vi "Mapping Data Plot.vi"() -> ()   [LabVIEW 2012]
uses:
  <vilib>/Utility/miscctls.llb/LVPointDoubleTypeDef.ctl
  <vilib>/Utility/file.llb/Write To Spreadsheet File (DBL).vi
panel:
  in  "Write to file":bool
  out "Counts under curve":dbl[][](array[numeric])=[[0.0, 105.0, 108.0, 96.0, 96.0, 91.0, 85.0], [0.0, 133.0, 105.0, 97.0, 115.0, 96.0, 86.0], [0.0, 257.0, 244.0, 227.0, 195.0, 194.0, 94.0], [0.0, 255.0, 253.0, 258.0, 293.0, 296.0, 96.0], [0.0, 125.0, 160.0, 164.0, 196.0, 206.0, 83.0], [0.0, 107.0, 106.0, 102.0, 94.0, 103.0, 99.0]]
  in  "Cursor.Cursor Position 2":T1
  in  "peak centerRcm-1":dbl=519.0
  in  "peak widthRcm-1":dbl=8.0
  out "error out":errorcluster
  out "Raman Map":dbl[][](graph)
  in  "stop":bool
  out "plot graph":cluster{"Y":dbl[], "Y":dbl[]}[](graph)
  in  "Path":path=path "E:/Documents/lab/Maps"
  in  "2 Letter File Name":string="QS"
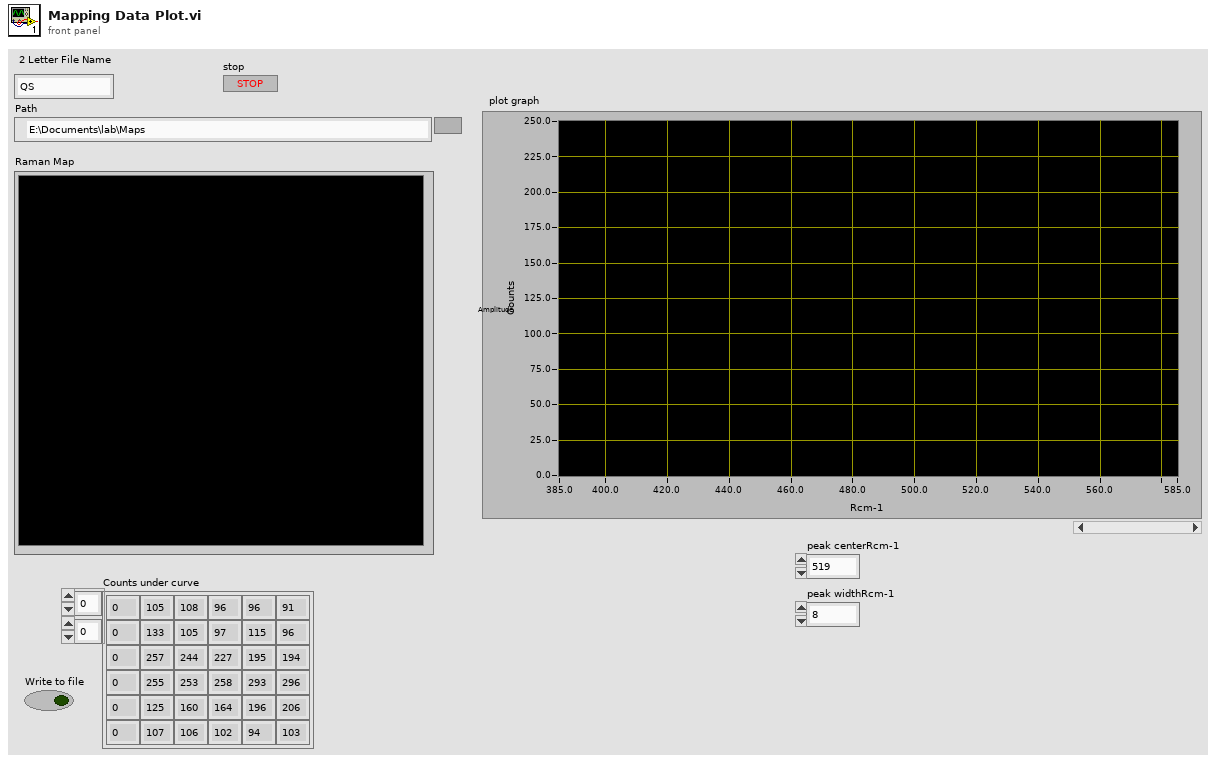
[diagram p1: front panel]
types:
  T1 = typedef "LVPointDoubleTypeDef.ctl" = cluster{"X":dbl, "Y":dbl}
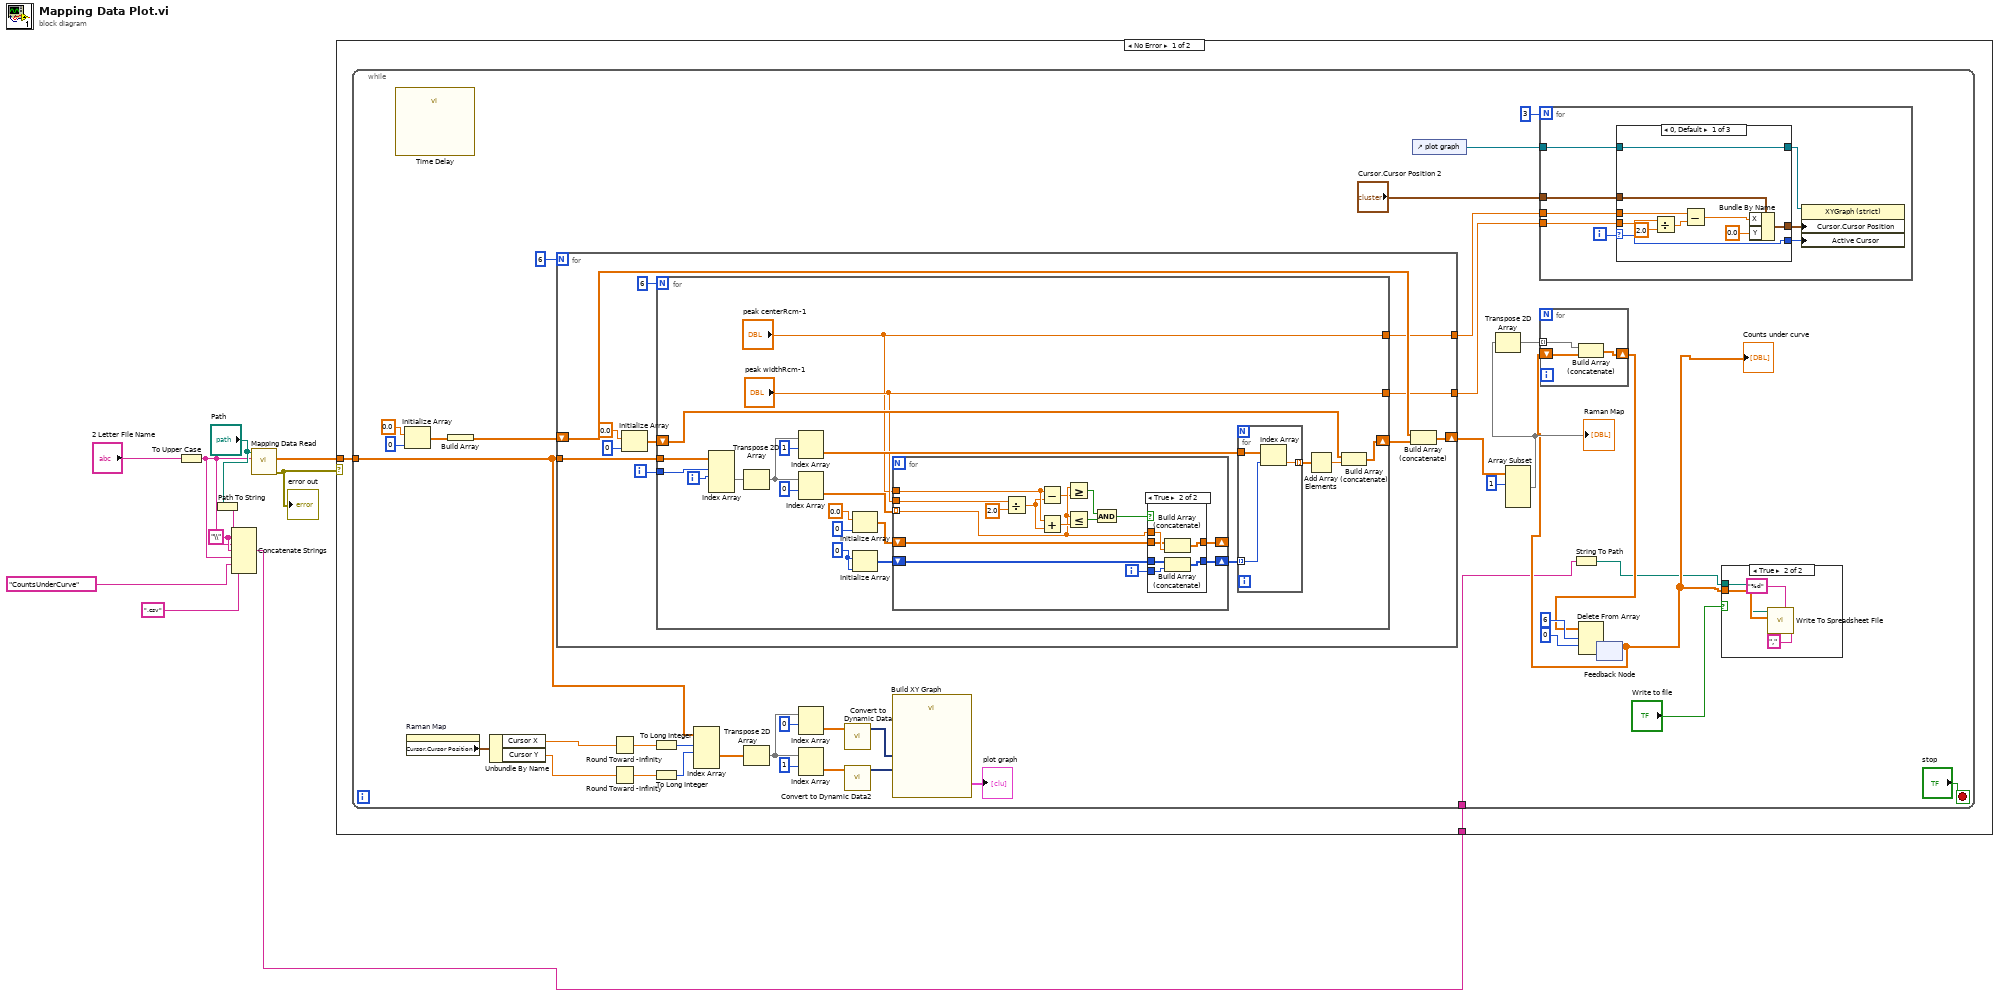
[diagram p0: block diagram]
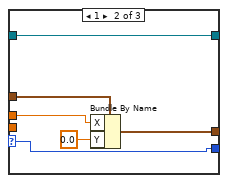
[diagram p3: hidden frame]
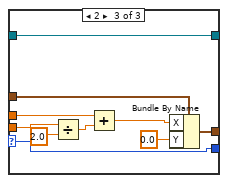
[diagram p4: hidden frame]
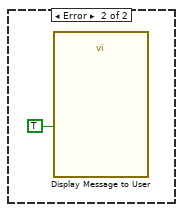
[diagram p6: hidden frame]
diagram:
  w5 = "\\" ("string")
  n1 = To Upper Case(1:"2 Letter File Name") -> (0:w3:string)
  n2 = Path To String(path="Path") -> (string=w6:string)
  n3 = Concatenate Strings(w6, w5, w3, w5, w3, "CountsUnderCurve" ("string"), ".csv") -> (w4:string)
  n4 = call "Mapping Data Read.vi"("Small File name"=w3, "Path"="Path") -> ("error out"=w9:errorcluster, "all rows"=w10:dbl[][][][])  [unwired: 8 in]
  "error out" <- w9
  n5 = case shown="No Error" w9 {
    tunnel: w10 -> [w12 _]
    tunnel: w4 -> [w11 _]
    frame No Error {
      n6 = while {
        tunnel: w12 -> [w43]
        tunnel: w11 -> [w15]
        stop <- "stop" stop-if-true
        n7 = call "Time Delay"() -> ()  [unwired: 11 in, 1 out]
        n8 = Initialize Array(0.0 ("element"), 0 ("dimension size")) -> (w39:dbl[])
        n9 = property on="Raman Map" class="IntGraph (strict)"() -> ("Cursor.Cursor Position"=w30:T1)  [unwired: 2 in, 2 out]
        n10 = Build Array(w39) -> (w38:dbl[][])
        n11 = Unbundle By Name(w30) -> ("Cursor X"=w22:dbl, "Cursor Y"=w29:dbl)
        n12 = for {
          N: 6 -> [_]
          tunnel: w43 -> [w104]
          shift-right: [w96] -> w24
          shift-left: w38 -> [w97]
          tunnel: [w95] -> w36
          tunnel: [w94] -> w32
          i -> [w103]
          n13 = Initialize Array(0.0 ("element"), 0 ("dimension size")) -> (w99:dbl[])
          n14 = for {
            N: 6 -> [_]
            tunnel: w104 -> [w116]
            tunnel: w103 -> [w115]
            shift-right: [w108] -> w98
            shift-left: w99 -> [w107]
            tunnel: ["peak centerRcm-1"] -> w95
            tunnel: ["peak widthRcm-1"] -> w94
            i -> [w110]
            w119 = 0 ("dimension size")
            n15 = Index Array(array=w116, index (dim 0)=w115, index (dim 1)=w110) -> (element=w117:dbl[][])  [unwired: 2 in]
            n16 = Transpose 2D Array(2D array=w117) -> (transposed array=w113:dbl[][])
            n17 = Index Array(array=w113, index (row)=1) -> (element=w111:dbl[])  [unwired: 1 in]
            n18 = Index Array(array=w113, index (row)=0) -> (element=w124:dbl[])  [unwired: 1 in]
            n19 = Initialize Array(0.0 ("element"), 0 ("dimension size")) -> (w122:dbl[])
            n20 = Initialize Array(w119, w119) -> (w120:i32[])
            n21 = for {
              tunnel: w124 -> [w139] mode=indexing
              shift-right: [w136] -> _
              shift-left: w122 -> [w137]
              shift-right: [w135] -> w114
              shift-left: w120 -> [w134]
              tunnel: "peak centerRcm-1" -> [w133]
              tunnel: "peak widthRcm-1" -> [w131]
              i -> [w138]
              n22 = Divide(x=w131, y=2.0) -> (x/y=w129:dbl)
              n23 = Subtract(x=w133, y=w129) -> (x-y=w130:dbl)
              n24 = Add(x=w133, y=w129) -> (x+y=w143:dbl)
              n25 = Greater Or Equal?(x=w139, y=w130) -> (x >= y?=w142:bool)
              n26 = Less Or Equal?(x=w139, y=w143) -> (x <= y?=w141:bool)
              n27 = And(x=w142, y=w141) -> (x .and. y?=w140:bool)
              n28 = case shown="True" w140 {
                tunnel: w139 -> [_ w151]
                tunnel: w138 -> [_ w148]
                tunnel: w137 -> [w145 w150]
                tunnel: [w145 w149] -> w136
                tunnel: [w144 w147] -> w135
                tunnel: w134 -> [w144 w146]
                frame False {
                }
                frame True {
                  n29 = Build Array (concatenate)(w150, w151) -> (w149:dbl[])
                  n30 = Build Array (concatenate)(w146, w148) -> (w147:i32[])
                }
              }
            }
            n31 = for {
              tunnel: w114 -> [w128] mode=indexing
              tunnel: [w127] -> w118 mode=indexing
              tunnel: w111 -> [w126]
              n32 = Index Array(array=w126, index=w128) -> (element=w127:dbl)
            }
            n33 = Add Array Elements(numeric array=w118) -> (sum=w109:dbl)
            n34 = Build Array (concatenate)(w107, w109) -> (w108:dbl[])
          }
          n35 = Build Array (concatenate)(w97, w98) -> (w96:dbl[][])
        }
        n36 = Round Toward -Infinity(1:w22) -> (0:w27:dbl)
        n37 = Round Toward -Infinity(1:w29) -> (0:w28:dbl)
        n38 = To Long Integer(number=w27) -> (32bit integer=w26:i32)
        n39 = To Long Integer(number=w28) -> (32bit integer=w25:i32)
        n40 = Index Array(array=w43, index (dim 0)=w26, index (dim 1)=w25) -> (element=w52:dbl[][])  [unwired: 2 in]
        n41 = Transpose 2D Array(2D array=w52) -> (transposed array=w51:dbl[][])
        n42 = Index Array(array=w51, index (row)=0) -> (element=w44:dbl[])  [unwired: 1 in]
        n43 = Index Array(array=w51, index (row)=1) -> (element=w41:dbl[])  [unwired: 1 in]
        n44 = call "Convert to Dynamic Data"("Array"=w44) -> ("Dynamic Data Type"=w47:dynamicdata)  [unwired: 3 in]
        n45 = call "Convert to Dynamic Data2"("Array"=w41) -> ("Dynamic Data Type"=w46:dynamicdata)  [unwired: 3 in]
        n46 = call "Build XY Graph"("Y Input"=w46, "X Input"=w47) -> ("XY Graph"=→"plot graph":cluster{"Y":dbl[], "Y":dbl[]}[])  [unwired: 3 in, 6 out]
        n47 = control-ref of="plot graph"() -> (w33:refnum<vi>)
        n48 = Array Subset(array=w24, index (row)=1 ("index")) -> (w21:dbl[][])  [unwired: 3 in]
        "Raman Map" <- w21
        n49 = Transpose 2D Array(2D array=w21) -> (transposed array=w31:dbl[][])
        n50 = for {
          N: 3 -> [_]
          tunnel: w36 -> [w60]
          tunnel: "Cursor.Cursor Position 2" -> [w66]
          tunnel: w33 -> [w65]
          tunnel: w32 -> [w64]
          i -> [w67]
          n51 = case shown="0, Default" w67 {
            selector: w67 -> [w76 w78 w92]
            tunnel: w60 -> [w70 w82 w87]
            tunnel: w66 -> [w74 w81 w90]
            tunnel: w65 -> [w77 w80 w93]
            tunnel: w64 -> [w71 _ w88]
            tunnel: [w77 w80 w93] -> w63
            tunnel: [w75 w79 w91] -> w62
            tunnel: [w76 w78 w92] -> w61
            frame 0, Default {
              n52 = Divide(x=w71, y=2.0) -> (x/y=w69:dbl)
              n53 = Subtract(x=w70, y=w69) -> (x-y=w68:dbl)
              n54 = Bundle By Name(cluster=w74, "X"=w68, "Y"=0.0) -> (w75:T1)
            }
            frame 1 {
              n55 = Bundle By Name(cluster=w81, "X"=w82, "Y"=0.0) -> (w79:T1)
            }
            frame 2 {
              n56 = Divide(x=w88, y=2.0) -> (x/y=w86:dbl)
              n57 = Add(x=w87, y=w86) -> (x+y=w85:dbl)
              n58 = Bundle By Name(cluster=w90, "X"=w85, "Y"=0.0) -> (w91:T1)
            }
          }
          n59 = property class="XYGraph (strict)"(reference=w63, "Cursor.Cursor Position"=w62, "Active Cursor"=w61) -> ()  [unwired: 1 in, 2 out]
        }
        n60 = String To Path(string=w15) -> (path=w14:path)
        n61 = feedback #1() -> (w16:dbl[][])  [unwired: 1 in]
        "Counts under curve" <- w16
        n62 = for {
          tunnel: w31 -> [w57] mode=indexing
          shift-right: [w59] -> w17
          shift-left: w16 -> [w58]
          n63 = Build Array (concatenate)(w57, w58) -> (w59:dbl[][])
        }
        n64 = Delete From Array(array=w17, length=6, index (row)=0) -> (deleted portion=w18:dbl[][])  [unwired: 1 in, 1 out]
        n65 = feedback-in #1(w18) -> ()
        n66 = case shown="True" "Write to file" {
          tunnel: w16 -> [_ w56]
          tunnel: w14 -> [_ w55]
          frame False {
          }
          frame True {
            n67 = call-poly <vilib>:"Write To Spreadsheet File.vi"("delimiter (\\t)"="," ("delimiter (\\t)"), "format (%.3f)"="%d", "2D data"=w56, "file path (dialog if empty)"=w55) -> ()  [unwired: 4 in, 1 out]
          }
        }
      }
    }
    frame Error {
      n68 = call "Display Message to User"("Enable"=TRUE) -> ()  [unwired: 9 in, 2 out]
    }
  }
